vi "FormatIncrementAction.vi"(1 "Limit action":T1) -> (0 "value":string)   [LabVIEW 2014, in "PythonConfiguration.lvclass"]
uses:
  PythonConfiguration.lvclass
  TypeDefs/IncrementAction.ctl
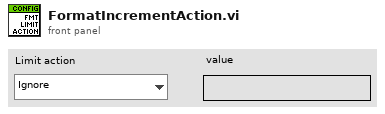
[diagram p1: front panel]
types:
  T1 = typedef "PythonConfiguration.lvclass/IncrementAction.ctl" = enum8{"Ignore", "Coerce to nearest", "Coerce up", "Coerce down"}
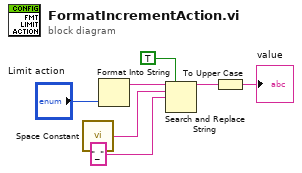
[diagram p0: block diagram]
diagram:
  n1 = call <vilib>:"Space Constant.vi"() -> ("String"=w2:string)
  n2 = Format Into String("Limit action") -> (resulting string=w5:string)  [unwired: 3 in, 1 out]
  n3 = Search and Replace String(replace all?=TRUE ("replace all? (F)"), input string=w5, search string=w2, replace string="_" ("replace string (\"\")")) -> (result string=w4:string)  [unwired: 4 in, 3 out]
  n4 = To Upper Case(1:w4) -> (0:→"value":string)
